vi "RP calculate subset PD.vi"(5 "Samples per trigger increment":i32=2, 6 "Round off":i32=1024 format="0x%x (%d)", 7 "RAM size":i32=268435456 format="0x%x (%d)", 8 "Trigger start position":i32 format="0x%x (%d)", 9 "Pre-trigger samples":i32=125000 format="0x%x (%d)", 10 "Bytes per sample":i32=4, 11 "Post-trigger samples":i32=50000000 format="0x%x (%d)") -> (0 "Merged subsets":u64[](array[numeric]) format="0x%x (%d)", 1 "record length":i32 format="0x%x (%d)", 2 "pre-trigger trim":i32 format="0x%x (%d)", 3 "Subsets":i32[][](array[numeric]) format="0x%x (%d)")   [LabVIEW 2024]
uses:
  Mode.ctl
panel:
  out "RAM locations":i32[][](array[numeric]) format="0x%x (%d)"
  out "end_pos":i32 format="0x%x (%d)"
  out "start_pos":i32 format="0x%x (%d)"
  out "actual trigger pos":i32 format="0x%x (%d)"
  out "unsigned 64bit integer":u64[](array[numeric]) format="%x"
  out "x << y":u64 format="%x"
  out "post-trigger trim":i32
  out "subset length":i32 format="0x%x (%d)"
  out "subset start":i32 format="0x%x (%d)"
  in  "Mode":T1=enum."Digitizer"
  # "ends"
  # "starts"
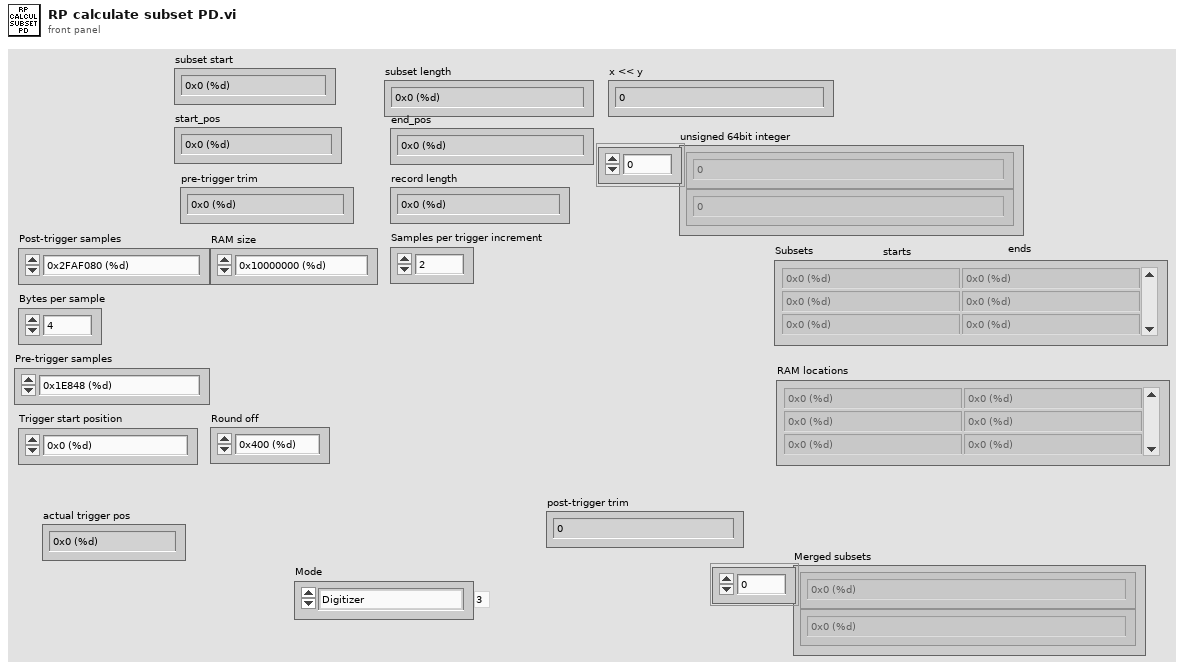
[diagram p1: front panel]
types:
  T1 = typedef "Mode.ctl" = enum16{"Filter", "Lockin test", "Snapshot test", "Digitizer", "Current-Voltage"}
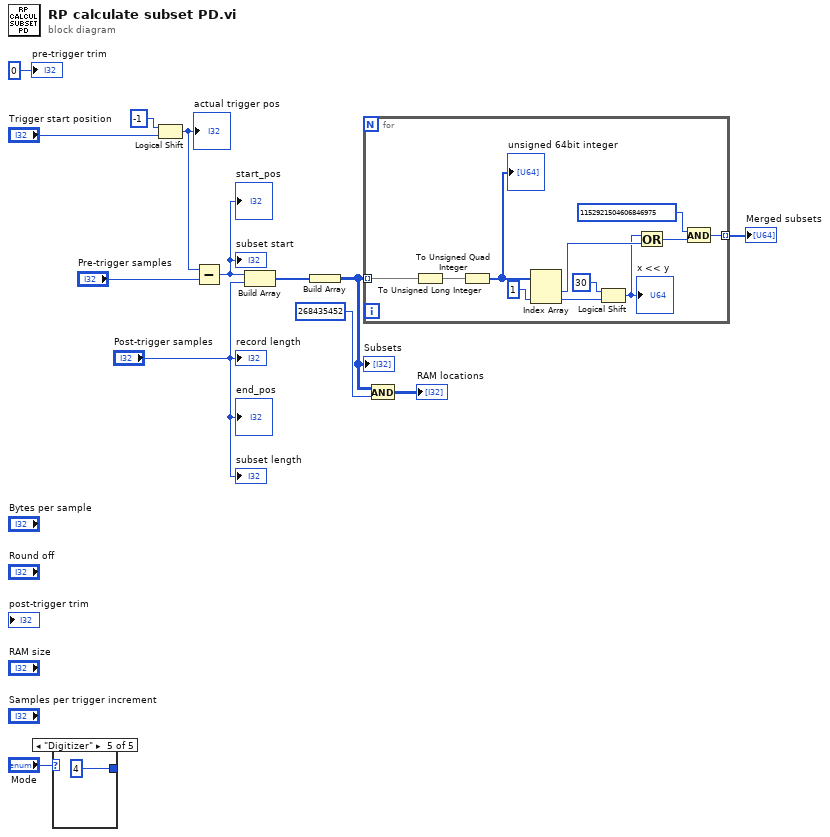
[diagram p0: block diagram]
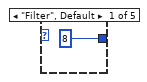
[diagram p2: hidden frame]
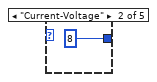
[diagram p3: hidden frame]
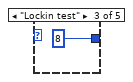
[diagram p4: hidden frame]
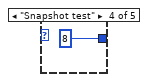
[diagram p5: hidden frame]
diagram:
  n1 = case shown="\"Digitizer\"" "Mode" {
    tunnel: [8 8 8 8 4] -> _
    frame "Filter", Default {
    }
    frame "Current-Voltage" {
    }
    frame "Lockin test" {
    }
    frame "Snapshot test" {
    }
    frame "Digitizer" {
    }
  }
  n2 = Logical Shift(y=i16 -1, x="Trigger start position") -> (x << y=w3:i32)
  "actual trigger pos" <- w3
  n3 = Subtract(x=w3, y="Pre-trigger samples") -> (x-y=w8:i32)
  "subset start" <- w8
  "start_pos" <- w8
  n4 = Build Array(w8, "Post-trigger samples") -> (w12:i32[])
  n5 = Build Array(w12) -> (w6:i32[][])
  "Subsets" <- w6
  n6 = for {
    tunnel: w6 -> [w29] mode=indexing
    tunnel: [w21] -> w10 mode=indexing
    n7 = To Unsigned Long Integer(number=w29) -> (unsigned 32bit integer=w19:u32[])
    n8 = To Unsigned Quad Integer(1:w19) -> (0:w28:u64[])
    "unsigned 64bit integer" <- w28
    n9 = Index Array(array=w28, index #2=1 ("index")) -> (element #1=w24:u64, element #2=w26:u64)  [unwired: 1 in]
    n10 = Logical Shift(y=i16 30, x=w26) -> (x << y=w23:u64)
    "x << y" <- w23
    n11 = Or(x=w23, y=w24) -> (x .or. y?=w22:u64)
    n12 = And(x=u64 1152921504606846975 ("value"), y=w22) -> (x .and. y?=w21:u64)
  }
  "Merged subsets" <- w10
  n13 = And(x=w6, y=268435452) -> (x .and. y?=→"RAM locations":i32[][])
  "pre-trigger trim" <- 0 ("pre-trigger trim")
  "subset length" <- "Post-trigger samples"
  "record length" <- "Post-trigger samples"
  "end_pos" <- "Post-trigger samples"
